vi "Clip AO Waveforms.vi"(8 "error in (no error)":errorcluster, 10 "AO []":waveform(dbl)[](array[waveform]), 11 "AO Configuration":T1 {"output terminal configuration" items=["Default"=-1, "RSE"=10083, "Differential"=10106, "Pseudodifferential"=12529]}) -> (0 "error out":errorcluster, 2 "Clipped AO []":waveform(dbl)[](array[waveform]))   [LabVIEW 2019, in "LockinDAQ.lvclass"]
uses:
  LockinDAQ.lvclass
  Instrument.Lockin/Instrument.Lockin.lvclass
  Typedefs/446xAO-enum.ctl
  Typedefs/DAQType-enum.ctl
  Typedefs/AO.config-cluster.ctl
  Typedefs/AO.config-array.ctl
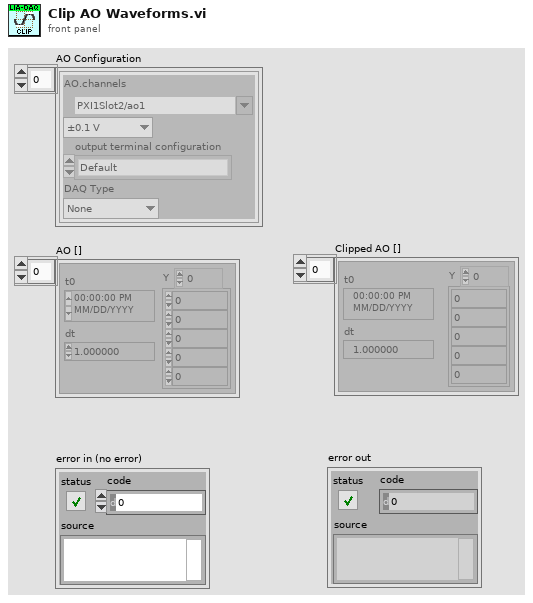
[diagram p1: front panel]
types:
  T1 = typedef "LockinDAQ.lvclass/AO.config-array.ctl" = T2[]
  T2 = typedef "LockinDAQ.lvclass/AO.config-cluster.ctl" = cluster{"AO.channels":tag, "AO.Range":T3, "output terminal configuration":i32, "DAQ Type":T4}
  T3 = typedef "LockinDAQ.lvclass/446xAO-enum.ctl" = enum16{"±0.1 V", "±1.0 V", "±10.0 V"}
  T4 = typedef "LockinDAQ.lvclass/DAQType-enum.ctl" = enum16{"None", "USB 4431", "PXI 446x"}
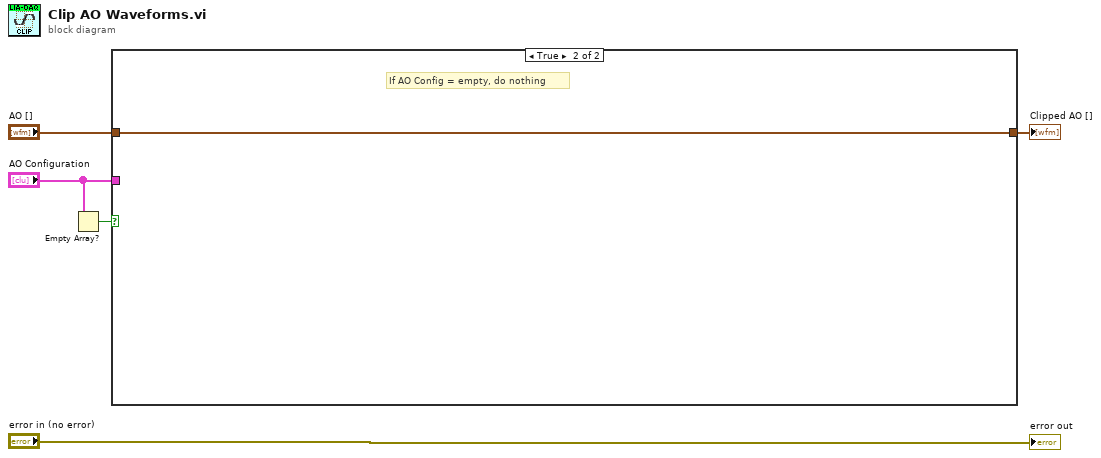
[diagram p0: block diagram]
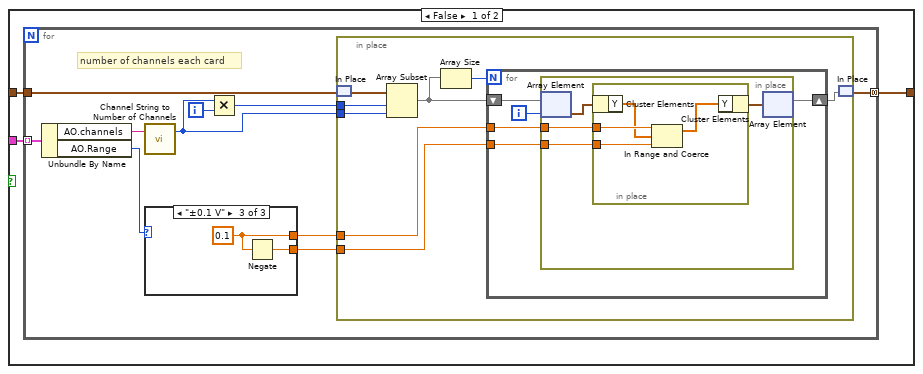
[diagram p2: hidden frame]
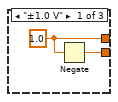
[diagram p3: hidden frame]
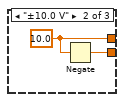
[diagram p4: hidden frame]
diagram:
  n1 = Empty Array?(array="AO Configuration") -> (empty?=w1:bool)
  n2 = case shown="True" w1 {
    tunnel: [w8 w46] -> w5
    tunnel: "AO []" -> [w7 w46]
    tunnel: "AO Configuration" -> [w6 _]
    frame False {
      n3 = for {
        tunnel: w6 -> [w16] mode=indexing
        tunnel: w7 -> [w9]
        tunnel: [w10] -> w8 mode=concatenating
        i -> [w15]
        # "number of channels each card"
        n4 = Unbundle By Name(w16) -> ("AO.channels"=w12:tag, "AO.Range"=w11:T3)
        n5 = call "Channel String to Number of Channels.vi"("Channels String"=w12) -> ("# channels"=w18:i32)  [unwired: 2 in]
        n6 = case shown="\"±0.1 V\"" w11 {
          tunnel: [w41 w43 w45] -> w14
          tunnel: [w40 w42 w44] -> w13
          frame "±1.0 V" {
            w41 = 1.0
            n7 = Negate(x=w41) -> (-x=w40:dbl)
          }
          frame "±10.0 V" {
            w43 = 10.0
            n8 = Negate(x=w43) -> (-x=w42:dbl)
          }
          frame "±0.1 V" {
            w45 = 0.1
            n9 = Negate(x=w45) -> (-x=w44:dbl)
          }
        }
        n10 = Multiply(x=w18, y=w15) -> (x*y=w17:i32)
        n11 = in-place {
          in-place-border: w18 -> [w26]
          in-place-border: w17 -> [w25]
          in-place-border: w14 -> [w24]
          in-place-border: w13 -> [w23]
          n12 = in-place-match #1(w9) -> (w22:waveform(dbl)[])
          n13 = Array Subset(array=w22, index=w25, length=w26) -> (w19:waveform(dbl)[])
          n14 = Array Size(array=w19) -> (size(s)=w20:i32)
          n15 = for {
            N: w20 -> [_]
            tunnel: w24 -> [w31]
            tunnel: w23 -> [w30]
            shift-right: [w27] -> w21
            shift-left: w19 -> [w28]
            i -> [w29]
            n16 = in-place {
              in-place-border: w31 -> [w35]
              in-place-border: w30 -> [w34]
              n17 = in-place-array #2(w28, w29) -> (w33:waveform(dbl))
              n18 = in-place {
                in-place-border: w35 -> [w39]
                in-place-border: w34 -> [w38]
                n19 = in-place-cluster #3(w33) -> ("Y"=w37:dbl[])
                n20 = In Range and Coerce(upper limit=w39, x=w37, lower limit=w38) -> (coerced(x)=w36:dbl[])  [unwired: 1 out]
                n21 = in-place-cluster #3("Y"=w36) -> (w32:waveform(dbl))
              }
              n22 = in-place-array #2(w32) -> (w27:waveform(dbl)[])  [unwired: 1 out]
            }
          }
          n23 = in-place-match #1(w21) -> (w10:waveform(dbl)[])
        }
      }
    }
    frame True {
      # "If AO Config = empty, do nothing"
    }
  }
  "Clipped AO []" <- w5
  "error out" <- "error in (no error)"
